vi "IVandLVManualtrace.vi"() -> ()   [LabVIEW 2020]
uses:
  <vilib>/MakerHub/LINX/Public/Peripherals/Analog/Analog Read 1 Chan.vi
  <vilib>/MakerHub/LINX/Public/Peripherals/Analog/Analog Read N Chans.vi
  <vilib>/MakerHub/LINX/Private/Local IO/LinxAnalogRead.vi
  <vilib>/MakerHub/LINX/Public/Utilities/Check Channel.vi
  <vilib>/MakerHub/LINX/Public/Utilities/Open Serial.vi
  <vilib>/MakerHub/LINX/Private/Utilties/Generate Error.vi
  <vilib>/Utility/file.llb/Write Delimited Spreadsheet (DBL).vi
  <vilib>/MakerHub/LINX/LMH-LINX.lvlib
panel:
  out "Light vs Voltage":cluster{"Y":dbl[], "Y":dbl[]}[](graph)
  in  "Record point":bool
  out "photodiode IV curve":cluster{"Y":dbl[], "Y":dbl[]}[](graph)
  out "?":dbl(graph)
  out "photodiode voltage":dbl(graph)
  out "Numeric":i32
  out "Error Out 2":errorcluster
  in  "stop":bool
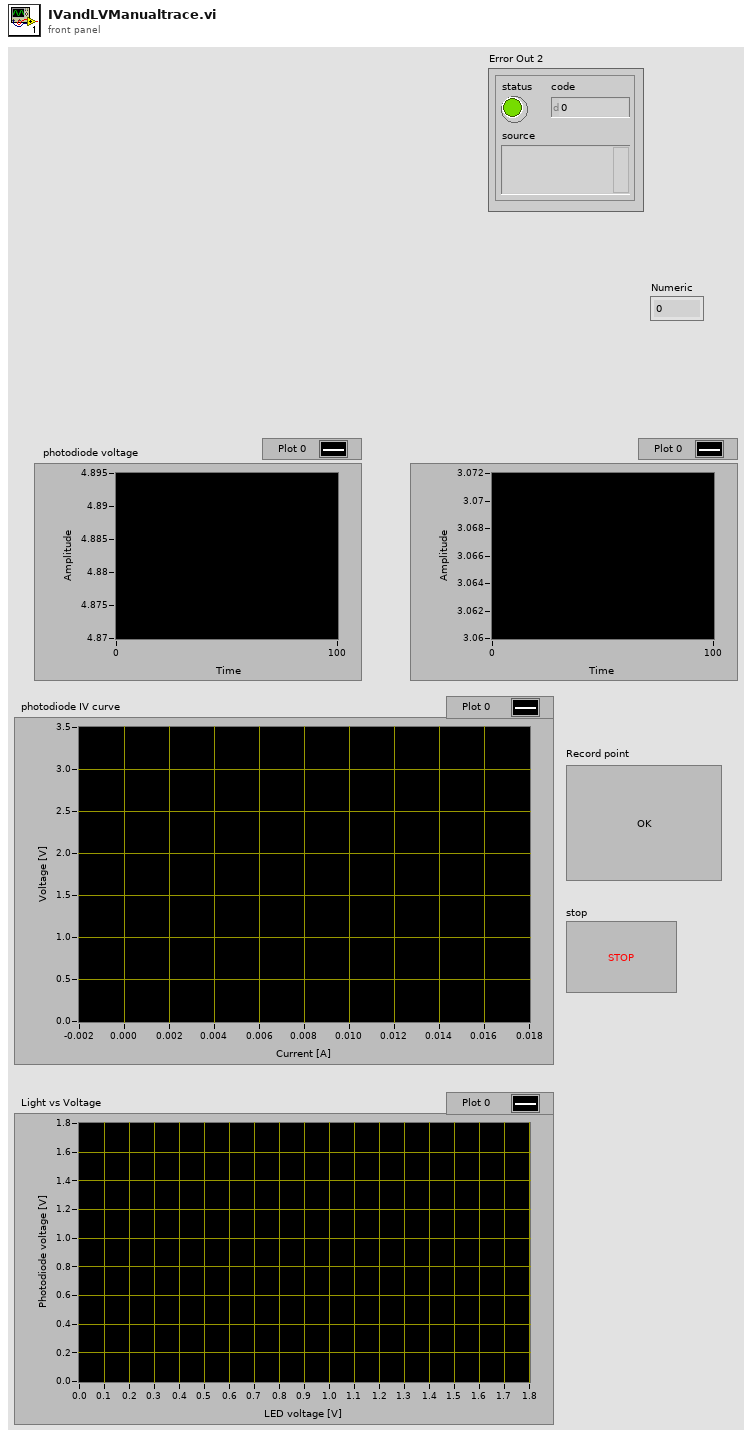
[diagram p1: front panel]
types:
  T1 = typedef "LMH-LINX.lvlib/LINX Ref.ctl" = cluster{"IO":T2, "Interface":T3, "LINX Device Config":T4}
  T2 = typedef "LMH-LINX.lvlib/Platform.ctl" = enum16{"Remote", "Local"}
  T3 = typedef "LMH-LINX.lvlib/Interface.ctl" = enum16{"Serial", "TCP"}
  T4 = typedef "LMH-LINX.lvlib/Device.lvlib/LINX Device Config.ctl" = cluster{"Interface":T3, "COM Port":refnum<visa-resource-name>, "TCP Configuration":T5, "Device Family":u8, "Device ID":u8, "Device Name":string, "TCP Ref":refnum<k5>, "Channels":T6}
  T5 = typedef "LMH-LINX.lvlib/Device.lvlib/TCP Config.ctl" = cluster{"IP Address":string, "Port":u16}
  T6 = typedef "LMH-LINX.lvlib/Channels.ctl" = cluster{"DI":u8[], "DO":u8[], "AI":u8[], "AO":u8[], "PWM":u8[], "QE":u8[], "UART":u8[], "I2C 2":u8[], "SPI":u8[], "CAN":u8[], "Servo":u8[], "AI Ref (V)":dbl, "AI Resolution (Bits)":u8, "AO Ref (V)":dbl, "AO Resolution (Bits)":u8}
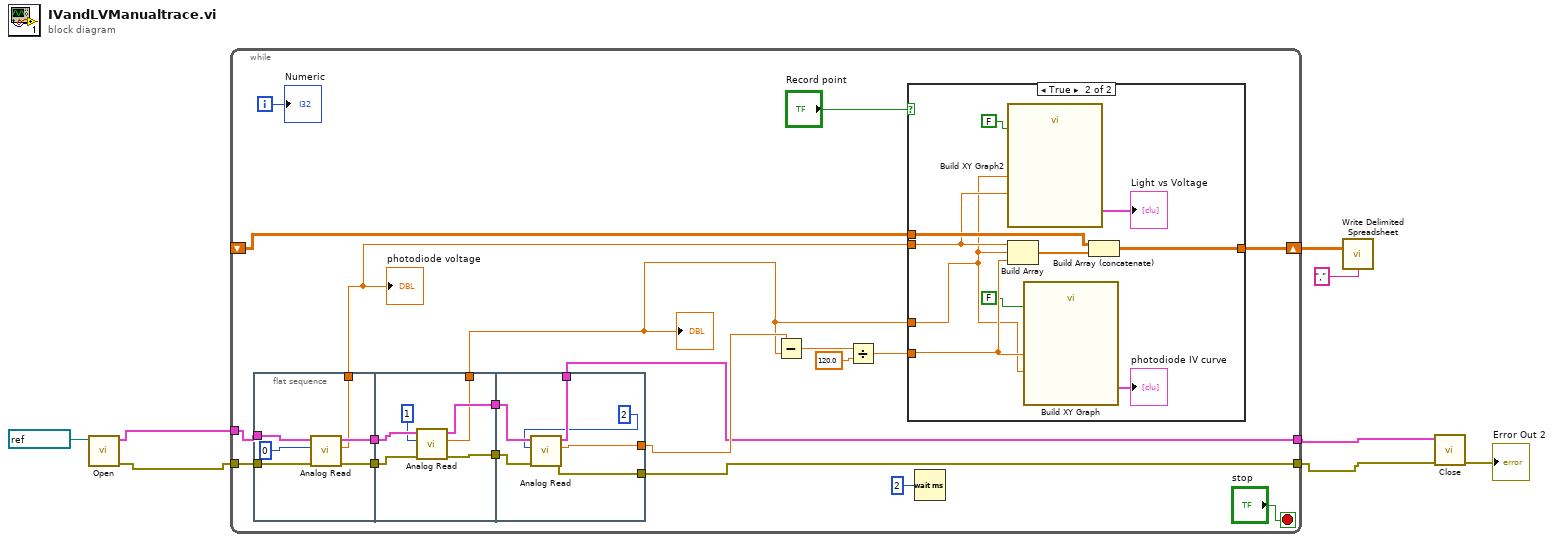
[diagram p0: block diagram]
diagram:
  n1 = call-poly <vilib>:"Open.vi"("Serial Port"=refnum<visa-resource-name> "COM4") -> ("Error Out"=w3:errorcluster, "LINX Resource"=w4:T1)  [unwired: 8 in, 1 out]
  n2 = while {
    tunnel: [w13] -> w2
    tunnel: [w11] -> w1
    shift-right: [w22] -> w6
    shift-left: _ -> [w23]
    tunnel: w3 -> [w19]
    tunnel: w4 -> [w18]
    i -> [w26]
    stop <- "stop" stop-if-true
    n3 = flat-sequence {
      tunnel: w19 -> [w31]
      tunnel: w18 -> [w30]
      tunnel: [w34] -> w17
      tunnel: [w33] -> w16
      tunnel: [w29] -> w10
      tunnel: w17 -> [w39]
      tunnel: w16 -> [w40]
      tunnel: [w38] -> w15
      tunnel: [w37] -> w14
      tunnel: [w35] -> w9
      tunnel: w15 -> [w46]
      tunnel: w14 -> [w45]
      tunnel: [w44] -> w13
      tunnel: [w43] -> w12
      tunnel: [w42] -> w11
      frame #0 {
        n4 = call-poly <vilib>:"Analog Read.vi"("Error In"=w31, "Analog Channel"=u8 0, "LINX Resource"=w30) -> ("Error Out"=w33:errorcluster, "Voltage"=w29:dbl, "LINX Resource"=w34:T1)  [unwired: 5 in, 1 out]
      }
      frame #1 {
        n5 = call-poly <vilib>:"Analog Read.vi"("Error In"=w40, "Analog Channel"=u8 1, "LINX Resource"=w39) -> ("Error Out"=w38:errorcluster, "Voltage"=w35:dbl, "LINX Resource"=w37:T1)  [unwired: 5 in, 1 out]
      }
      frame #2 {
        n6 = call-poly <vilib>:"Analog Read.vi"("Error In"=w46, "Analog Channel"=u8 2, "LINX Resource"=w45) -> ("Error Out"=w44:errorcluster, "Voltage"=w43:dbl, "LINX Resource"=w42:T1)  [unwired: 5 in, 1 out]
      }
    }
    n7 = Subtract(x=w12, y=w9) -> (x-y=w25:dbl)
    n8 = Divide(x=w25, y=120.0) -> (x/y=w21:dbl)
    n9 = case shown="True" "Record point" {
      tunnel: w23 -> [w47 w57]
      tunnel: [w47 w56] -> w22
      tunnel: w21 -> [_ w53]
      tunnel: w10 -> [_ w49]
      tunnel: w9 -> [_ w48]
      frame False {
      }
      frame True {
        n10 = call "Build XY Graph2"("Reset"=FALSE, "Y Input"=w49, "X Input"=w48) -> ("XY Graph"=→"Light vs Voltage":cluster{"X":dbl[], "Y":dbl[]}[])  [unwired: 7 in, 1 out]
        n11 = Build Array(w49, w48, w53) -> (w55:dbl[])
        n12 = call "Build XY Graph"("Reset"=FALSE, "Y Input"=w48, "X Input"=w53) -> ("XY Graph"=→"photodiode IV curve":cluster{"X":dbl[], "Y":dbl[]}[])  [unwired: 7 in, 1 out]
        n13 = Build Array (concatenate)(w57, w55) -> (w56:dbl[][])
      }
    }
    n14 = Wait (ms)(milliseconds to wait=u32 2) -> ()  [unwired: 1 out]
    "Numeric" <- w26
    "photodiode voltage" <- w10
    "?" <- w9
  }
  n15 = call-poly <vilib>:"Write Delimited Spreadsheet.vi"("2D data"=w6, "delimiter (\\t)"="," ("delimiter (\\t)")) -> ()  [unwired: 12 in, 2 out]
  n16 = call <vilib>:"Close.vi"("Error In"=w2, "LINX Resource"=w1) -> ("Error Out"=→"Error Out 2":errorcluster)  [unwired: 9 in]
